vi "RTS Update Values Both Save and No Save.vi"(0 "All Data":dbl[][](array[numeric]) format="%.6f", 5 "error in":errorcluster, 7 "Chamber 1 Socket":string[][](array[string]), 8 "Tree Selection":T1, 9 "Chamber 2 Socket":string[][](array[string]), 11 "Chamber 3 Socket":string[][](array[string]), 13 "Chamber 4 Socket":string[][](array[string])) -> (10 "Point File Name":string, 12 "Chamber Data":string[][](array[string]), 14 "Plot Data Array":dbl[][](array[numeric]) format="%.6f", 16 "Full Item Names":string[](array[string]), 17 "Listbox Data":string[][](array[string]), 18 "Custom Titles":string[](array[string]), 19 "error out":errorcluster)   [LabVIEW 2020]
uses:
  Type Definitions/RTS Room Selector.ctl
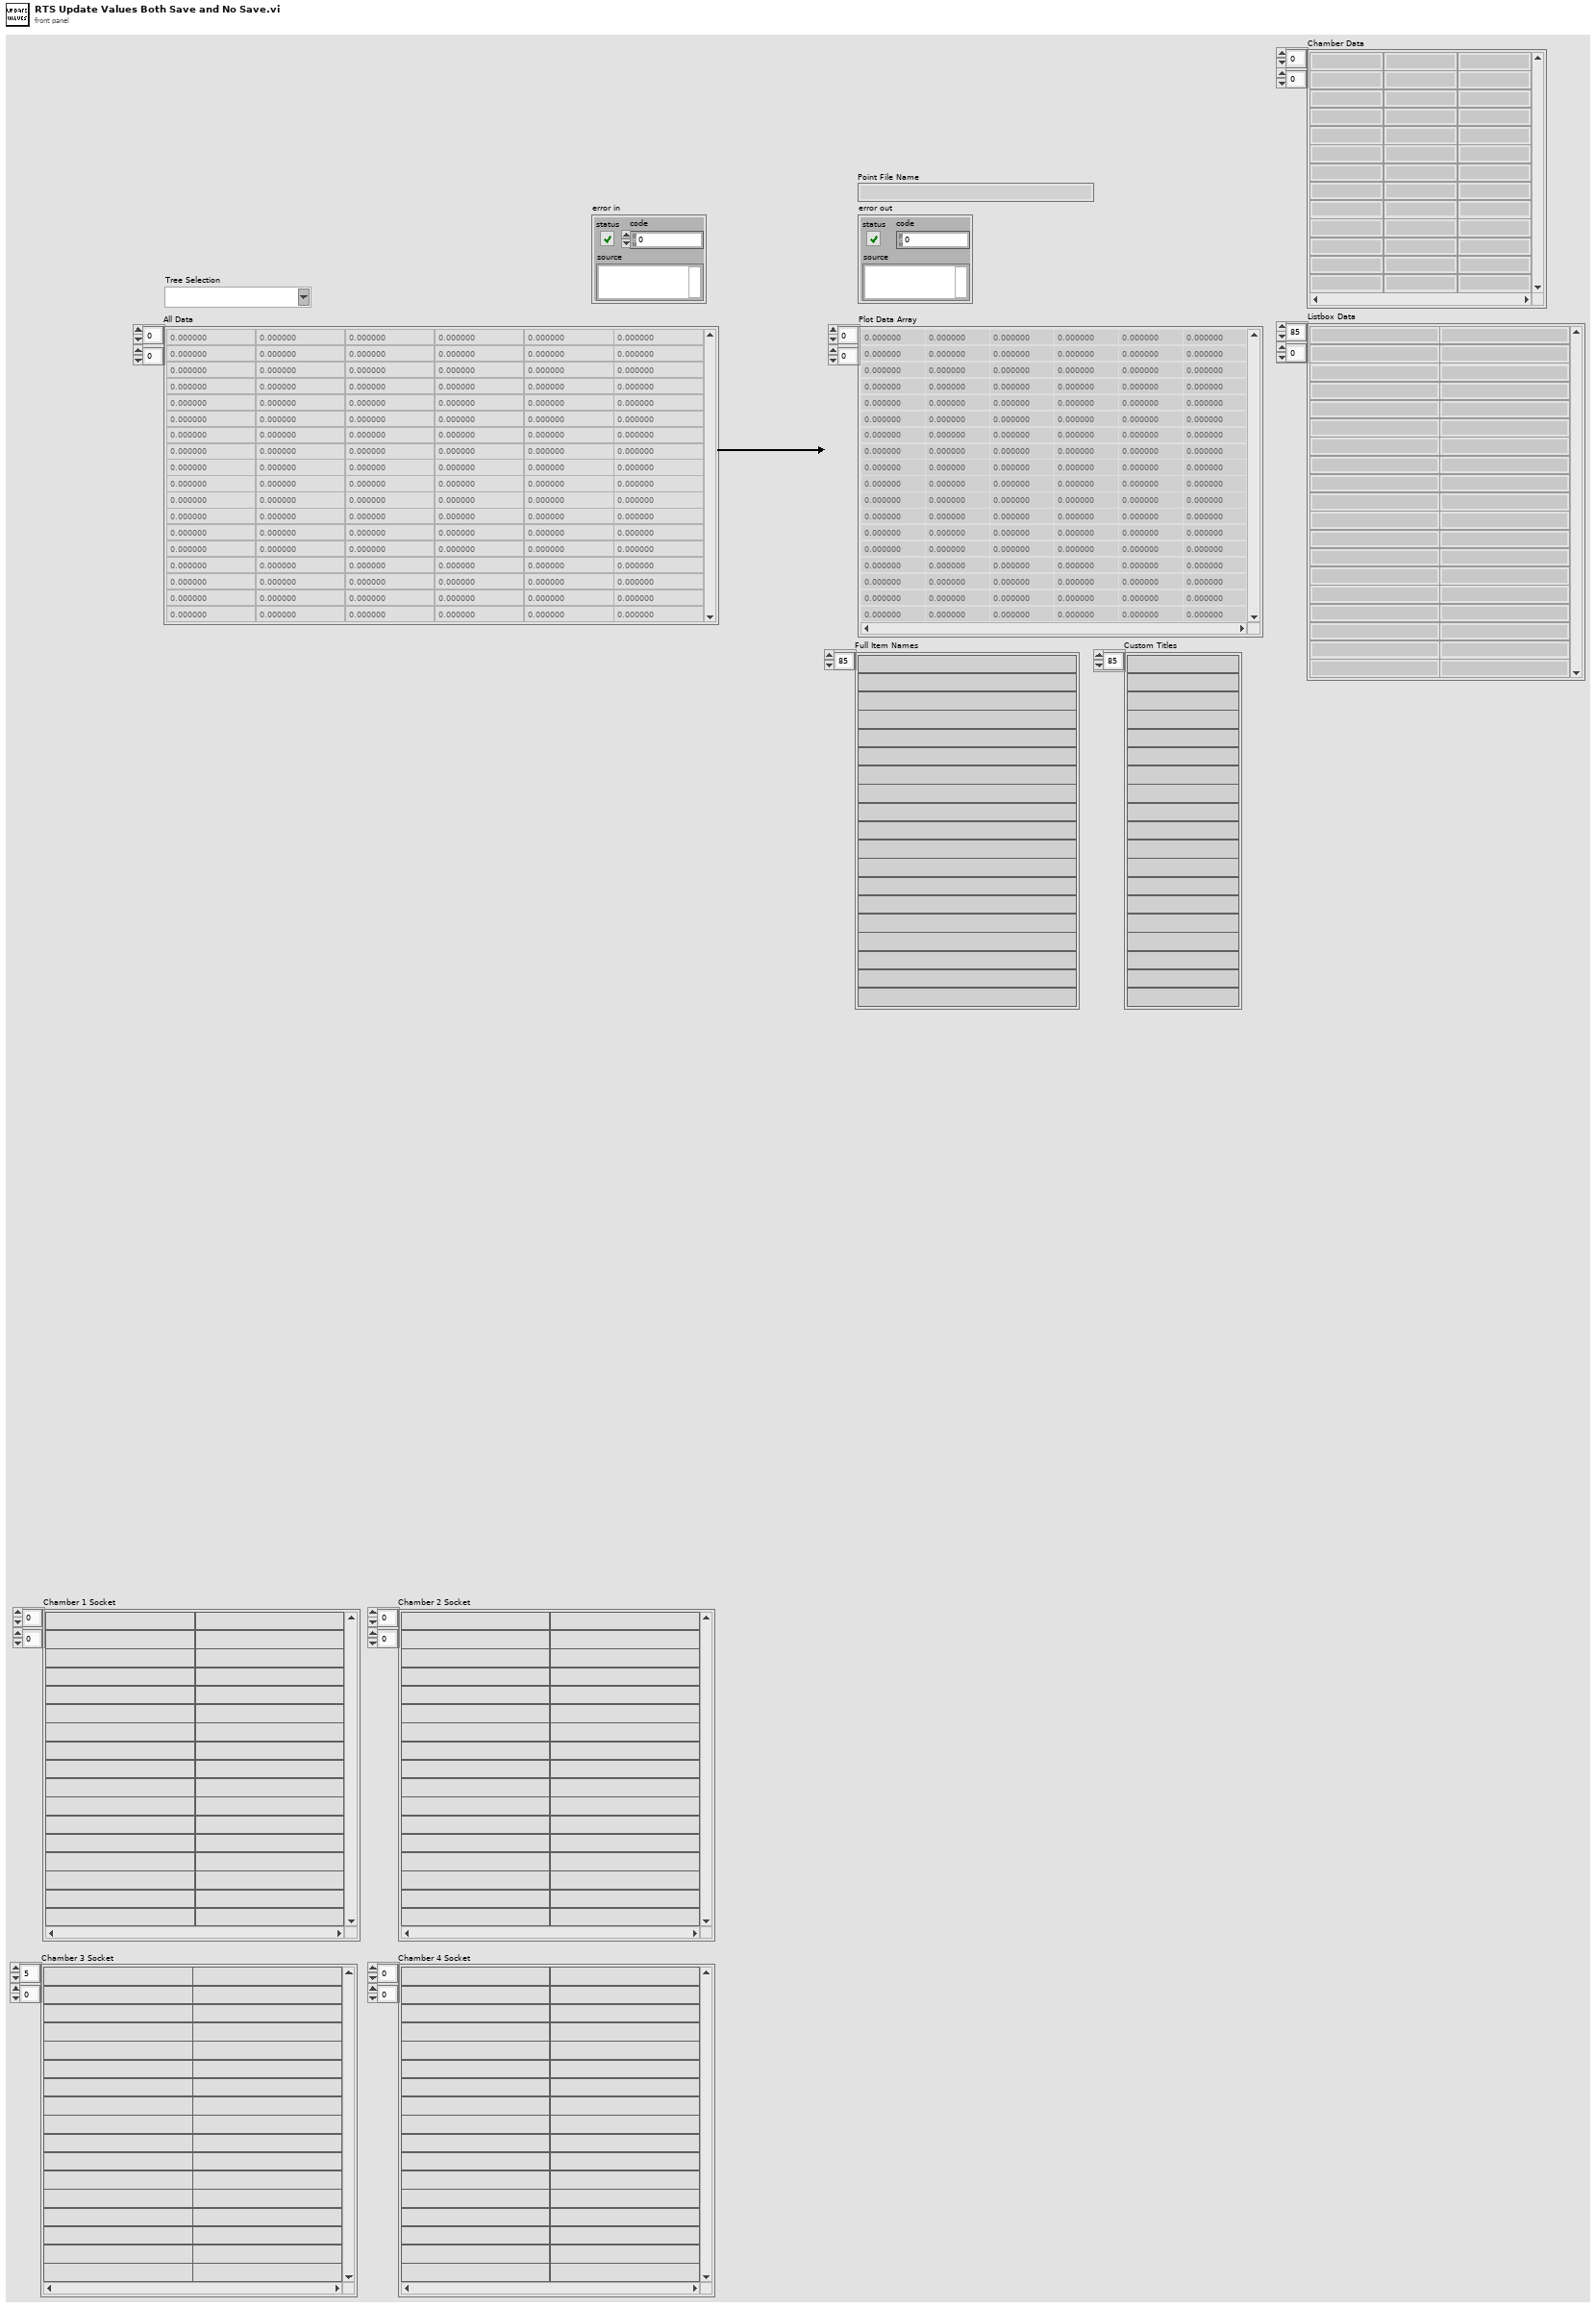
[diagram p1: front panel]
types:
  T1 = typedef "RTS Room Selector.ctl" = string
  T2 = typedef "RTS TDMS Data.ctl" = cluster{"Station 1":dbl[][], "Station 2":dbl[][], "Station 3":dbl[][], "Station 4":dbl[][], "Station 5":dbl[][], "Station 6":dbl[][], "Station 7":dbl[][], "Station 8":dbl[][]}
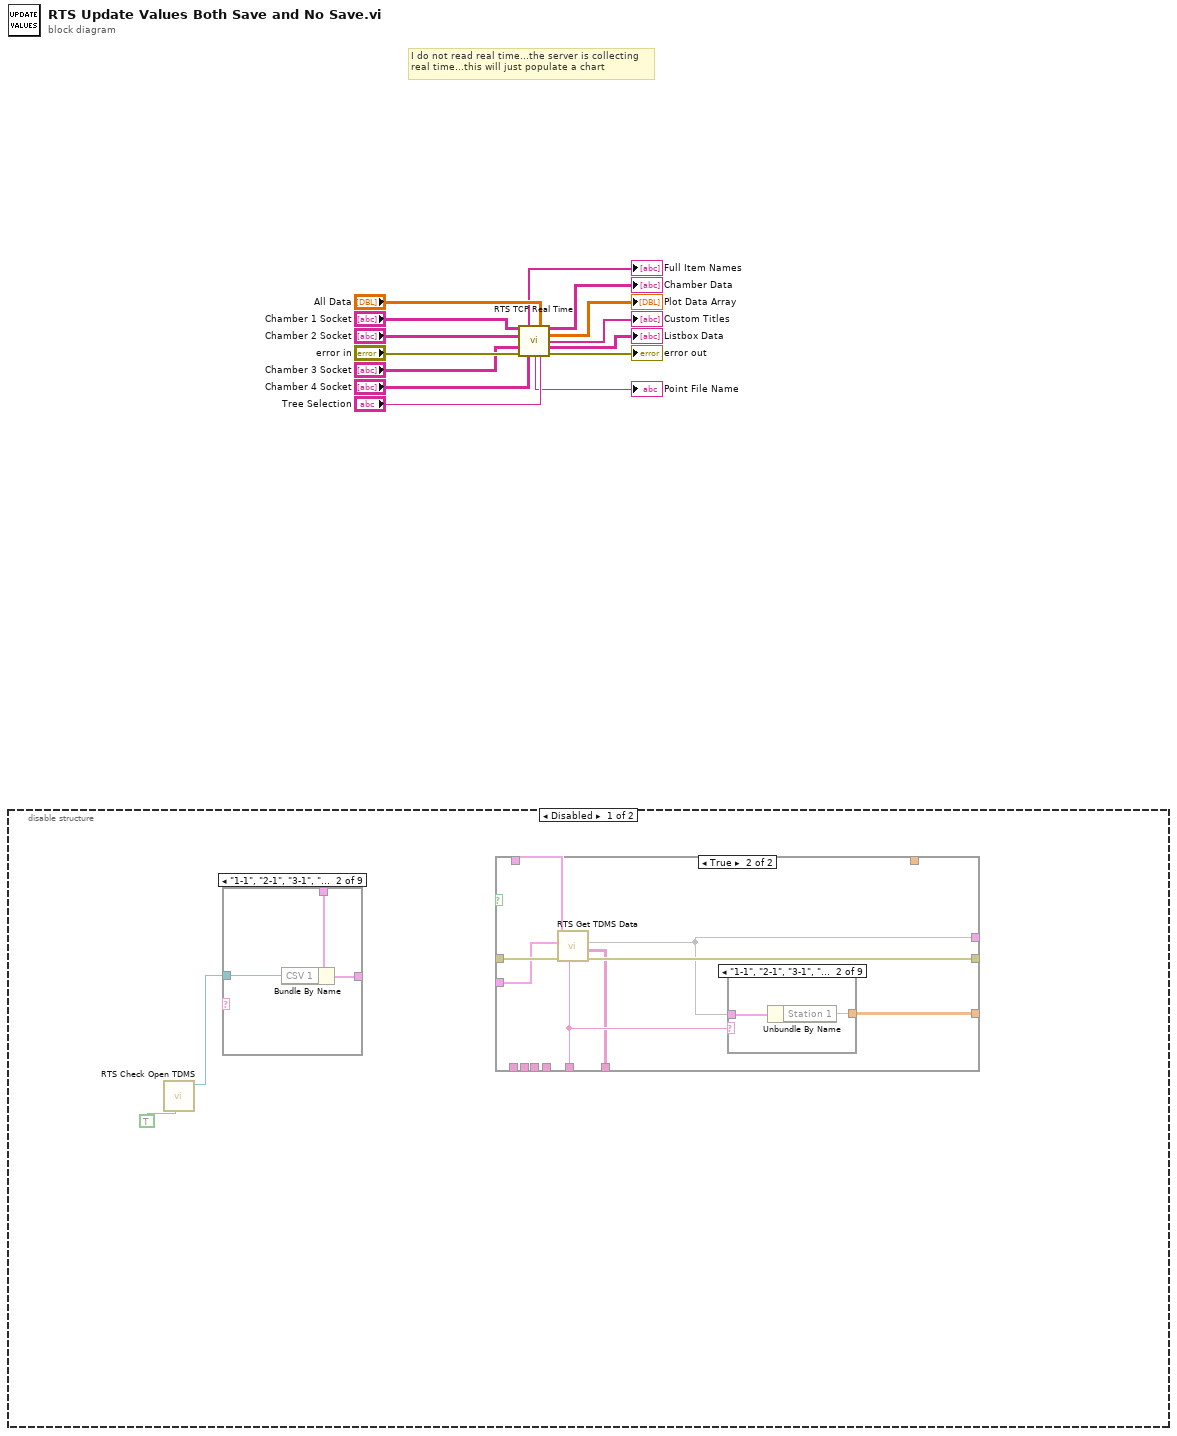
[diagram p0: block diagram]
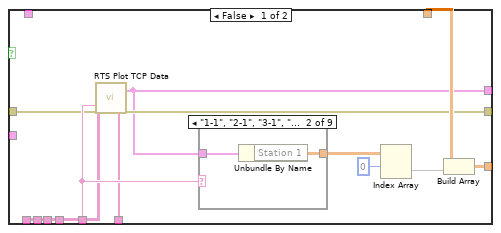
[diagram p2: hidden frame]
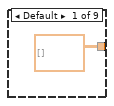
[diagram p3: hidden frame]
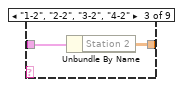
[diagram p4: hidden frame]
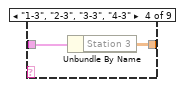
[diagram p5: hidden frame]
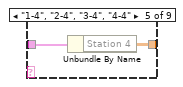
[diagram p6: hidden frame]
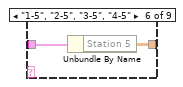
[diagram p7: hidden frame]
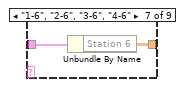
[diagram p8: hidden frame]
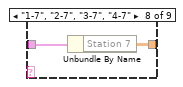
[diagram p9: hidden frame]
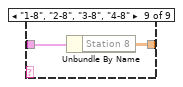
[diagram p10: hidden frame]
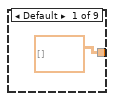
[diagram p11: hidden frame]
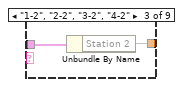
[diagram p12: hidden frame]
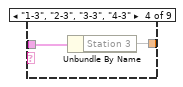
[diagram p13: hidden frame]
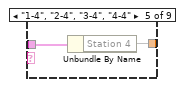
[diagram p14: hidden frame]
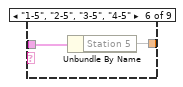
[diagram p15: hidden frame]
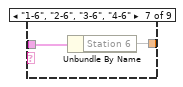
[diagram p16: hidden frame]
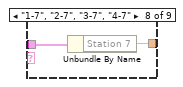
[diagram p17: hidden frame]
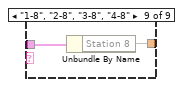
[diagram p18: hidden frame]
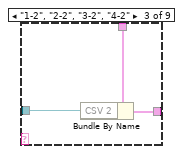
[diagram p20: hidden frame]
diagram:
  # "I do not read real time...the server is collecting\nreal time...this will just populate a chart"
  n1 = disable-structure shown="Disabled" {
    frame Disabled {
      n2 = call "RTS Check Open TDMS.vi"(6:TRUE ("Asy Read?")) -> ("error out"=w22:errorcluster, "Open All CSV Data"=w21:bool, "Byte Stream File Out"=w15:refnum<file>, "error in (no error)"=w16:errorcluster, "CSV File Location"=w17:path, "Byte Stream File In"=w23:refnum<file>)  [unwired: 5 in]
      n3 = case shown="\"1-1\", \"2-1\", \"3-1\", \"4-1\"" w20 {
        tunnel: [w80 w83 w86 w89 w92 w95 w98 w101 w104] -> w19
        tunnel: [w80 w81 w85 w88 w91 w94 w97 w100 w103] -> _
        tunnel: w15 -> [_ w82 w84 w87 w90 w93 w96 w99 w102]
        frame Default {
        }
        frame "1-1", "2-1", "3-1", "4-1" {
          n4 = Bundle By Name(cluster=w83, "CSV 1"=w82) -> (w81:cluster{})
        }
        frame "1-2", "2-2", "3-2", "4-2" {
          n5 = Bundle By Name(cluster=w86, "CSV 2"=w84) -> (w85:cluster{})
        }
        frame "1-3", "2-3", "3-3", "4-3" {
          n6 = Bundle By Name(cluster=w89, "CSV 3"=w87) -> (w88:cluster{})
        }
        frame "1-4", "2-4", "3-4", "4-4" {
          n7 = Bundle By Name(cluster=w92, "CSV 4"=w90) -> (w91:cluster{})
        }
        frame "1-5", "2-5", "3-5", "4-5" {
          n8 = Bundle By Name(cluster=w95, "CSV 5"=w93) -> (w94:cluster{})
        }
        frame "1-6", "2-6", "3-6", "4-6" {
          n9 = Bundle By Name(cluster=w98, "CSV 6"=w96) -> (w97:cluster{})
        }
        frame "1-7", "2-7", "3-7", "4-7" {
          n10 = Bundle By Name(cluster=w101, "CSV 7"=w99) -> (w100:cluster{})
        }
        frame "1-8", "2-8", "3-8", "4-8" {
          n11 = Bundle By Name(cluster=w104, "CSV 8"=w102) -> (w103:cluster{})
        }
      }
      n12 = case shown="True" {
        selector: _ -> [_ _]
        tunnel: [w25 w59] -> _
        tunnel: [w26 w61] -> _
        tunnel: _ -> [_ w60]
        tunnel: _ -> [w32 w58]
        tunnel: _ -> [w27 w62]
        tunnel: [w24 w55] -> _
        tunnel: [w35 w57] -> _
        tunnel: _ -> [w34 _]
        tunnel: _ -> [w31 _]
        tunnel: _ -> [w30 _]
        tunnel: _ -> [w29 _]
        tunnel: _ -> [w28 _]
        tunnel: _ -> [_ w56]
        frame False {
          n13 = call "RTS Plot TCP Data.vi"("Chamber 1 Socket"=w31, "Chamber 2 Socket"=w30, "Chamber 3 Socket"=w29, "Chamber 4 Socket"=w28, "Tree Selection in"=w32, "Error In"=w27) -> ("Full Item Names"=w24:string[], "CSV Data out"=w25:T2, "Error Out"=w26:errorcluster)  [unwired: 6 in, 5 out]
          n14 = case shown="\"1-1\", \"2-1\", \"3-1\", \"4-1\"" w32 {
            tunnel: [dbl[][] [] w40 w42 w44 w46 w48 w50 w52 w54] -> w33
            tunnel: w25 -> [_ w39 w41 w43 w45 w47 w49 w51 w53]
            frame Default {
            }
            frame "1-1", "2-1", "3-1", "4-1" {
              n15 = Unbundle By Name(w39) -> ("Station 1"=w40:dbl[][])
            }
            frame "1-2", "2-2", "3-2", "4-2" {
              n16 = Unbundle By Name(w41) -> ("Station 2"=w42:dbl[][])
            }
            frame "1-3", "2-3", "3-3", "4-3" {
              n17 = Unbundle By Name(w43) -> ("Station 3"=w44:dbl[][])
            }
            frame "1-4", "2-4", "3-4", "4-4" {
              n18 = Unbundle By Name(w45) -> ("Station 4"=w46:dbl[][])
            }
            frame "1-5", "2-5", "3-5", "4-5" {
              n19 = Unbundle By Name(w47) -> ("Station 5"=w48:dbl[][])
            }
            frame "1-6", "2-6", "3-6", "4-6" {
              n20 = Unbundle By Name(w49) -> ("Station 6"=w50:dbl[][])
            }
            frame "1-7", "2-7", "3-7", "4-7" {
              n21 = Unbundle By Name(w51) -> ("Station 7"=w52:dbl[][])
            }
            frame "1-8", "2-8", "3-8", "4-8" {
              n22 = Unbundle By Name(w53) -> ("Station 8"=w54:dbl[][])
            }
          }
          n23 = Index Array(array=w33, index (row)=0) -> (element=w36:dbl[])  [unwired: 1 in]
          n24 = Build Array(w34, w36) -> (w35:dbl[][])
        }
        frame True {
          n25 = call "RTS Get TDMS Data.vi"("Tree Selection"=w58, "error in (no error)"=w62, 10:w60, "CSV Data Save"=w56) -> ("error out"=w61:errorcluster, "Listbox names"=w55:string[][], 2:w59)  [unwired: 4 in, 1 out]
          n26 = case shown="\"1-1\", \"2-1\", \"3-1\", \"4-1\"" w58 {
            tunnel: [dbl[][] [] w65 w67 w69 w71 w73 w75 w77 w79] -> w57
            tunnel: w59 -> [_ w64 w66 w68 w70 w72 w74 w76 w78]
            frame Default {
            }
            frame "1-1", "2-1", "3-1", "4-1" {
              n27 = Unbundle By Name(w64) -> ("Station 1"=w65)
            }
            frame "1-2", "2-2", "3-2", "4-2" {
              n28 = Unbundle By Name(w66) -> ("Station 2"=w67)
            }
            frame "1-3", "2-3", "3-3", "4-3" {
              n29 = Unbundle By Name(w68) -> ("Station 3"=w69)
            }
            frame "1-4", "2-4", "3-4", "4-4" {
              n30 = Unbundle By Name(w70) -> ("Station 4"=w71)
            }
            frame "1-5", "2-5", "3-5", "4-5" {
              n31 = Unbundle By Name(w72) -> ("Station 5"=w73)
            }
            frame "1-6", "2-6", "3-6", "4-6" {
              n32 = Unbundle By Name(w74) -> ("Station 6"=w75)
            }
            frame "1-7", "2-7", "3-7", "4-7" {
              n33 = Unbundle By Name(w76) -> ("Station 7"=w77)
            }
            frame "1-8", "2-8", "3-8", "4-8" {
              n34 = Unbundle By Name(w78) -> ("Station 8"=w79)
            }
          }
        }
      }
    }
    frame Enabled {
    }
  }
  n35 = call "RTS TCP Real Time.vi"("Chamber 1 Socket"="Chamber 1 Socket", "All Data in"="All Data", "Chamber 2 Socket"="Chamber 2 Socket", "Chamber 3 Socket"="Chamber 3 Socket", "error in (no error)"="error in", "Chamber 4 Socket"="Chamber 4 Socket", "Tree Selection"="Tree Selection") -> ("Full Item Names"=→"Full Item Names":string[], "Chamber Data"=→"Chamber Data":string[][], "All Data out"=→"Plot Data Array":dbl[][], "Custom Titles"=→"Custom Titles":string[], "Listbox Data"=→"Listbox Data":string[][], "Point File Name"=→"Point File Name":string, "error out"=→"error out":errorcluster)  [unwired: 2 in]
